vi "Symphony Client.vi"() -> ()   [LabVIEW 2019]
panel:
  in  "Write":bool
  in  "stop":bool
  in  "SympClient":cluster{"Message":string, "Data":variant, i32}={"Message"="InitCam", "Data"=variant, 0}
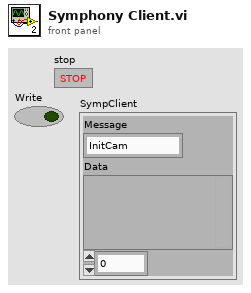
[diagram p1: front panel]
types:
  T1 = enum16{"Read", "Write", "ReadWrite", "BufferedRead", "BufferedReadWrite"}
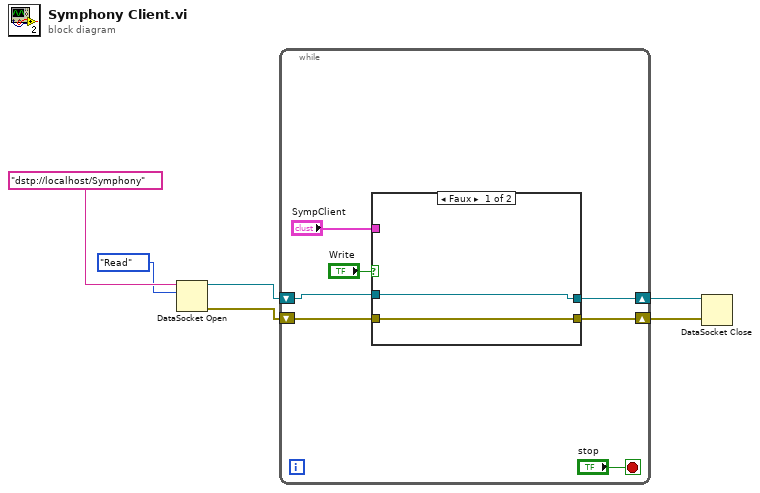
[diagram p0: block diagram]
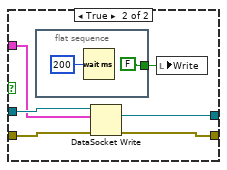
[diagram p2: hidden frame]
diagram:
  n1 = DataSocket Open(10:T1."Read" ("mode"), 11:"dstp://localhost/Symphony" ("URL")) -> (0:w2:errorcluster, 3:w1:refnum<k13>)  [unwired: 2 in]
  n2 = while {
    shift-right: [w12] -> w4
    shift-left: w2 -> [w7]
    shift-right: [w11] -> w3
    shift-left: w1 -> [w8]
    stop <- "stop" stop-if-true
    n3 = case shown="Faux" "Write" {
      tunnel: w8 -> [w15 w21]
      tunnel: "SympClient" -> [_ w17]
      tunnel: w7 -> [w14 w20]
      tunnel: [w14 w19] -> w12
      tunnel: [w15 w18] -> w11
      frame False {
      }
      frame True {
        n4 = flat-sequence {
          tunnel: [FALSE] -> w16
          frame #0 {
            n5 = Wait (ms)(milliseconds to wait=u32 200) -> ()  [unwired: 1 out]
          }
        }
        n6 = DataSocket Write(8:w20, 10:w17, 11:w21) -> (0:w19:errorcluster, 3:w18:refnum<k13>)  [unwired: 1 in, 1 out]
        n7 = local write "Write"(w16) -> ()
      }
    }
  }
  n8 = DataSocket Close(8:w4, 11:w3) -> ()  [unwired: 1 in, 2 out]
